vi "Get Attribute DBL.vi"(8 "error in":errorcluster, 10 "Attribute":string, 11 "IConfigurable in":refnum<class "IConfigurable.lvclass">) -> (0 "error out":errorcluster, 2 "Value":dbl, 3 "IConfigurable out":refnum<class "IConfigurable.lvclass">)   [LabVIEW 2024, in "IConfigurable.lvclass"]
uses:
  IConfigurable.lvclass
  IConfigure/IConfigure.lvclass
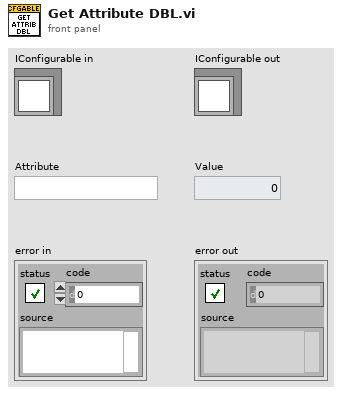
[diagram p1: front panel]
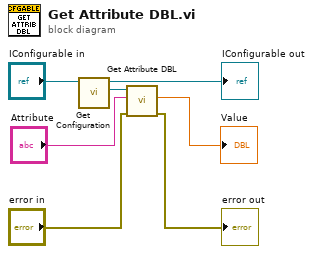
[diagram p0: block diagram]
diagram:
  n1 = call-dynamic "Get Configuration.vi"("IConfigurable in"="IConfigurable in") -> ("IConfigure.lvclass"=w5:refnum<class "IConfigure.lvclass">, "IConfigurable out"=→"IConfigurable out":refnum<class "IConfigurable.lvclass">)  [unwired: 9 in]
  n2 = call-dynamic "Get Attribute DBL.vi"("error in"="error in", "Attribute"="Attribute", "IConfigure in"=w5) -> ("error out"=→"error out":errorcluster, "Value"=→"Value":dbl)  [unwired: 6 in, 1 out]
